vi "DetectExtendCollision.vi"(4 "Ball":T1, 5 "Goal":dbl[](array[numeric]), 6 "Robot in":T2={"id"=0, "function"=enum."Attacker", "x"=0.0, "y"=0.0, "orientation"=0.0, "v_tangent"=0.0, "v_normal"=0.0, "v_ang"=0.0, "kick_x"=0.0, "kick_z"=0.0, "dribble"=FALSE, "Timestamp"=timestamp(0 s since 1904-01-01), "estimatives"={"est_v_tangent"=0.0, "est_v_normal"=0.0, "est_vx"=0.0, "est_vy"=0.0, "Pos Robot Est"=[]}, "dest_x_kick"=0.0, "dest_y_kick"=0.0, "Gap Coord"=[], "States"=enum."GoToTangent", "Path "=[], "Path  Smooth"=[], "Dest"=[], "vx_desired"=0.0, "vy_desired"=0.0}, 7 "Initial State":dbl[](array[numeric]), 9 "enemy_robots":T2[](array[typedef]), 10 "Point":dbl[](array[numeric]), 11 "our_robots":T2[](array[typedef])) -> (2 "Collision":bool)   [LabVIEW 2018]
uses:
  Vision_class/Old vision/Controls/AI Robot.ctl
  Vision_class/Old vision/Controls/Functions Enum.ctl
  Vision_class/Old vision/Controls/AttackerStates.ctl
  Vision_class/Old vision/Controls/PathDests.ctl
  Vision_class/Old vision/Controls/PathDest.ctl
  Communication_class/Paths/MessageAI_State Folder/Core/AI Ball.ctl
  Utilities_class/Utilities.lvclass
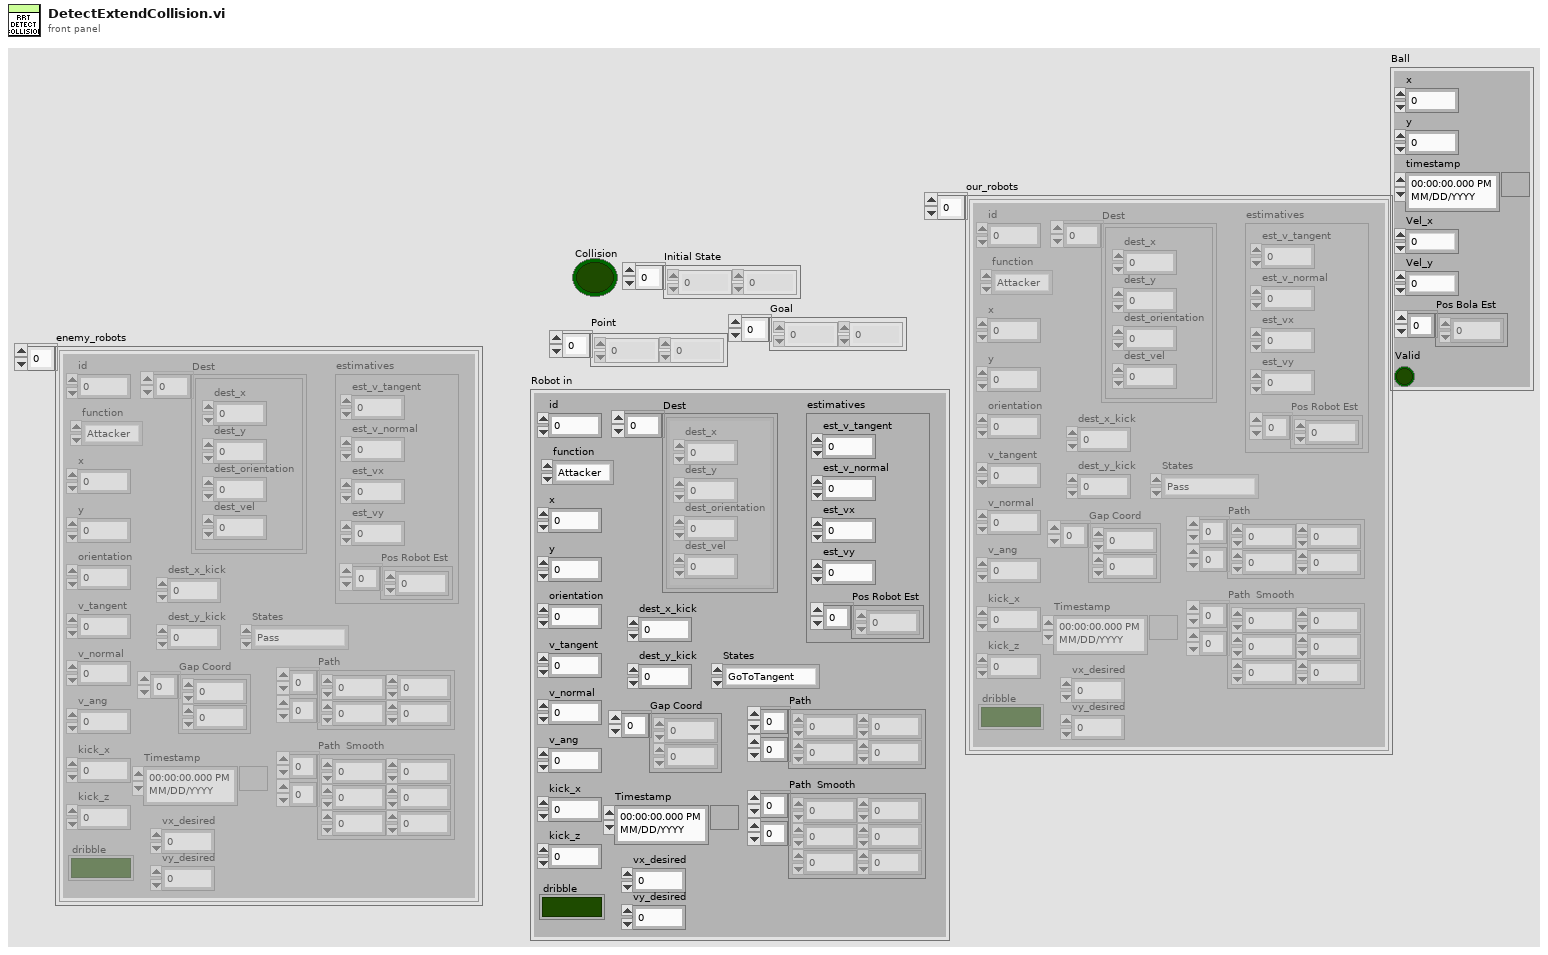
[diagram p1: front panel]
types:
  T1 = typedef "AI Ball.ctl" = cluster{"x":dbl, "y":dbl, "timestamp":timestamp, "Vel_x":dbl, "Vel_y":dbl, "Pos Bola Est":dbl[], "Valid":bool}
  T2 = typedef "AI Robot.ctl" = cluster{"id":u32, "function":T3, "x":dbl, "y":dbl, "orientation":dbl, "v_tangent":dbl, "v_normal":dbl, "v_ang":dbl, "kick_x":dbl, "kick_z":dbl, "dribble":bool, "Timestamp":timestamp, "estimatives":cluster{"est_v_tangent":dbl, "est_v_normal":dbl, "est_vx":dbl, "est_vy":dbl, "Pos Robot Est":dbl[]}, "dest_x_kick":dbl, "dest_y_kick":dbl, "Gap Coord":dbl[], "States":T4, "Path ":dbl[][], "Path  Smooth":dbl[][], "Dest":T5, "vx_desired":dbl, "vy_desired":dbl}
  T3 = typedef "Functions Enum.ctl" = enum16{"2nd Striker", "Attacker", "Goalie", "Defender", "Striker", "Goto 0", "Dummy", "Kicker", "ZigZag 0", "ZigZag 1", "ZigZag 2", "ZigZag 3", "ZigZag 4", "ZigZag 5", "ZigZag 6", "ZigZag 7", "ZigZag 8", ""}
  T4 = typedef "AttackerStates.ctl" = enum16{"Pass", "GoToTangent", "BallGetting", "GoToKick", ""}
  T5 = typedef "PathDests.ctl" = T6[]
  T6 = typedef "PathDest.ctl" = cluster{"dest_x":dbl, "dest_y":dbl, "dest_orientation":dbl, "dest_vel":dbl}
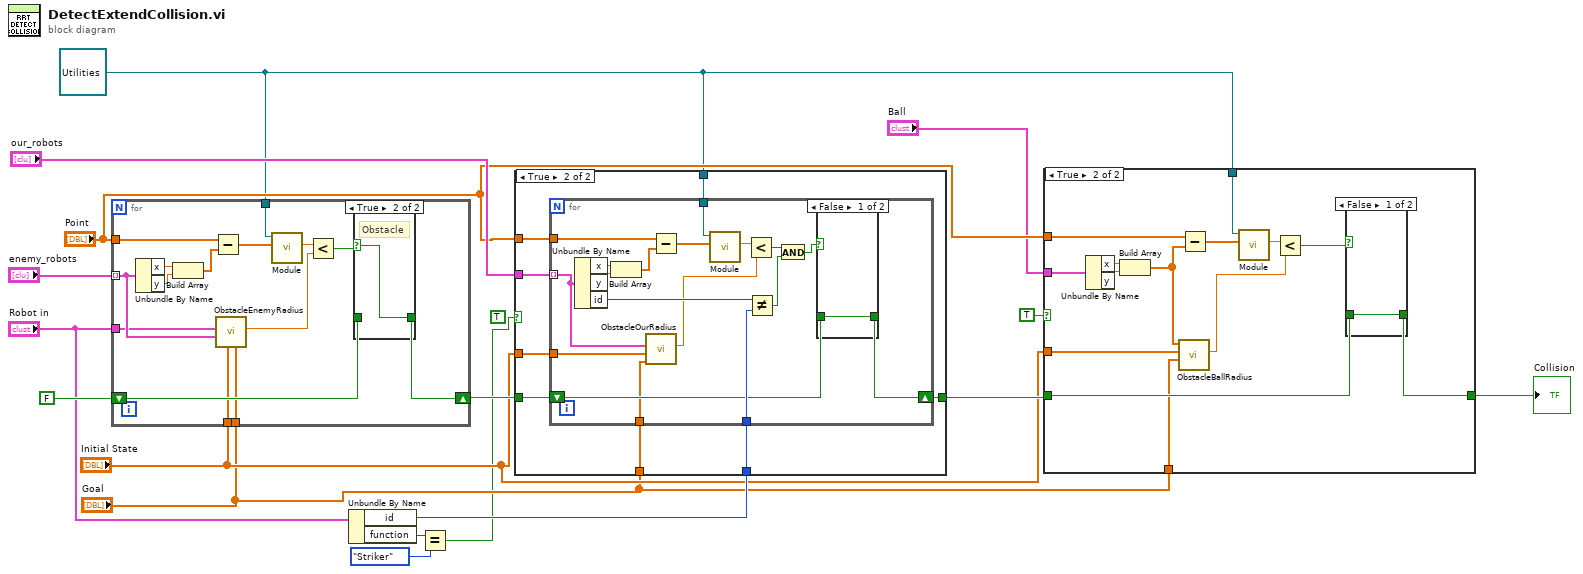
[diagram p0: block diagram]
diagram:
  w1 = refnum<class "Utilities.lvclass"> refnum ("Utilities in")
  (unwired) TRUE
  n1 = for {
    tunnel: "enemy_robots" -> [w22] mode=indexing
    tunnel: "Point" -> [w29]
    shift-right: [w24] -> w12
    shift-left: FALSE -> [w25]
    tunnel: "Robot in" -> [w21]
    tunnel: "Initial State" -> [w20]
    tunnel: "Goal" -> [w19]
    tunnel: w1 -> [w18]
    n2 = Unbundle By Name(w22) -> ("x"=w32:dbl, "y"=w31:dbl)
    n3 = Build Array(w32, w31) -> (w30:dbl[])
    n4 = Subtract(x=w29, y=w30) -> (x-y=w28:dbl[])
    n5 = call "ObstacleEnemyRadius.vi"("Goal"=w19, "Initial State"=w20, "Robot enemy"=w22, "Robot in"=w21) -> ("obstacle enemy radius"=w23:dbl)  [unwired: 7 in]
    n6 = call-dynamic "Module.vi"("2D vector"=w28, "Utilities in"=w18) -> ("Modulo"=w27:dbl)  [unwired: 7 in, 2 out]
    n7 = Less?(x=w27, y=w23) -> (x < y?=w26:bool)
    n8 = case shown="True" w26 {
      selector: w26 -> [_ w34]
      tunnel: w25 -> [w33 _]
      tunnel: [w33 w34] -> w24
      frame False {
      }
      frame True {
        # "Obstacle"
      }
    }
  }
  n9 = Unbundle By Name("Robot in") -> ("id"=w13:u32, "function"=w4:T3)
  n10 = Equal?(x=w4, y=Functions_Enum."Striker") -> (x = y?=w2:bool)
  n11 = case shown="True" w2 {
    tunnel: w12 -> [w35 w43]
    tunnel: "our_robots" -> [_ w42]
    tunnel: "Point" -> [_ w41]
    tunnel: [w35 w40] -> w9
    tunnel: w13 -> [_ w39]
    tunnel: "Initial State" -> [_ w38]
    tunnel: "Goal" -> [_ w37]
    tunnel: w1 -> [_ w36]
    frame False {
    }
    frame True {
      n12 = for {
        tunnel: w42 -> [w45] mode=indexing
        tunnel: w41 -> [w58]
        shift-right: [w55] -> w40
        shift-left: w43 -> [w49]
        tunnel: w39 -> [w50]
        tunnel: w38 -> [w47]
        tunnel: w37 -> [w46]
        tunnel: w36 -> [w44]
        n13 = Unbundle By Name(w45) -> ("x"=w61:dbl, "y"=w60:dbl, "id"=w51:u32)
        n14 = Build Array(w61, w60) -> (w59:dbl[])
        n15 = call "ObstacleOurRadius.vi"("Goal"=w46, "Initial State"=w47, "other robot"=w45) -> ("obstacle enemy radius"=w48:dbl)  [unwired: 8 in]
        n16 = Subtract(x=w58, y=w59) -> (x-y=w57:dbl[])
        n17 = call-dynamic "Module.vi"("2D vector"=w57, "Utilities in"=w44) -> ("Modulo"=w56:dbl)  [unwired: 7 in, 2 out]
        n18 = Less?(x=w56, y=w48) -> (x < y?=w54:bool)
        n19 = Not Equal?(x=w51, y=w50) -> (x != y?=w52:bool)
        n20 = And(x=w54, y=w52) -> (x .and. y?=w53:bool)
        n21 = case shown="False" w53 {
          selector: w53 -> [_ w63]
          tunnel: w49 -> [w62 _]
          tunnel: [w62 w63] -> w55
          frame False {
          }
          frame True {
            # "Obstacle"
          }
        }
      }
    }
  }
  n22 = case shown="True" TRUE {
    tunnel: w9 -> [w64 w78]
    tunnel: "Ball" -> [_ w77]
    tunnel: "Point" -> [_ w76]
    tunnel: [w64 w75] -> w11
    tunnel: "Initial State" -> [_ w68]
    tunnel: "Goal" -> [_ w67]
    tunnel: w1 -> [_ w65]
    frame False {
    }
    frame True {
      n23 = Unbundle By Name(w77) -> ("x"=w71:dbl, "y"=w70:dbl)
      n24 = Build Array(w71, w70) -> (w69:dbl[])
      n25 = call "ObstacleBallRadius.vi"("Goal"=w67, "Initial State"=w68, "ball"=w69) -> ("obstacle enemy radius"=w66:dbl)  [unwired: 8 in]
      n26 = Subtract(x=w76, y=w69) -> (x-y=w74:dbl[])
      n27 = call-dynamic "Module.vi"("2D vector"=w74, "Utilities in"=w65) -> ("Modulo"=w73:dbl)  [unwired: 7 in, 2 out]
      n28 = Less?(x=w73, y=w66) -> (x < y?=w72:bool)
      n29 = case shown="False" w72 {
        selector: w72 -> [_ w80]
        tunnel: w78 -> [w79 _]
        tunnel: [w79 w80] -> w75
        frame False {
        }
        frame True {
          # "Obstacle"
        }
      }
    }
  }
  "Collision" <- w11
